vi "MGCC_FntStaMach_figureplot_main.vi"() -> ()   [LabVIEW 2016]
doc: "-----------------------------------------------------------------------------------------------------------------------\nCopyright <2019> <The University of Tennessee at Knoxville and the University of Tennessee Research Foundation>\nThis software is released under BSD-3 \nhttps://opensource.org/licenses/BSD-3-Clause \nAdditional license options available at https://utrf.tennessee.edu/industry/sample-agreements/\n-----------------------------------------------------------------------------------------------------------------------"
panel:
  out "Voltage difference1 14":cluster{dbl[], dbl[]}(graph)
  out "Voltage difference1 13":cluster{dbl[], dbl[]}(graph)
  out "Voltage difference1 11":cluster{dbl[], dbl[]}(graph)
  out "Voltage difference1 10":cluster{dbl[], dbl[]}(graph)
  out "Voltage difference1 9":cluster{dbl[], dbl[]}(graph)
  out "Voltage difference1 8":cluster{dbl[], dbl[]}(graph)
  out "Voltage difference1 7":cluster{dbl[], dbl[]}(graph)
  out "Voltage difference1 6":cluster{dbl[], dbl[]}(graph)
  out "Voltage difference1 5":cluster{dbl[], dbl[]}(graph)
  out "Voltage difference1 4":cluster{dbl[], dbl[]}(graph)
  out "Voltage difference1 3":cluster{dbl[], dbl[]}(graph)
  out "Voltage difference1 2":cluster{dbl[], dbl[]}(graph)
  out "Voltage phase":cluster{dbl[], dbl[]}[](graph)
  out "Voltage difference1":cluster{dbl[], dbl[]}(graph)
  # "Voltage"
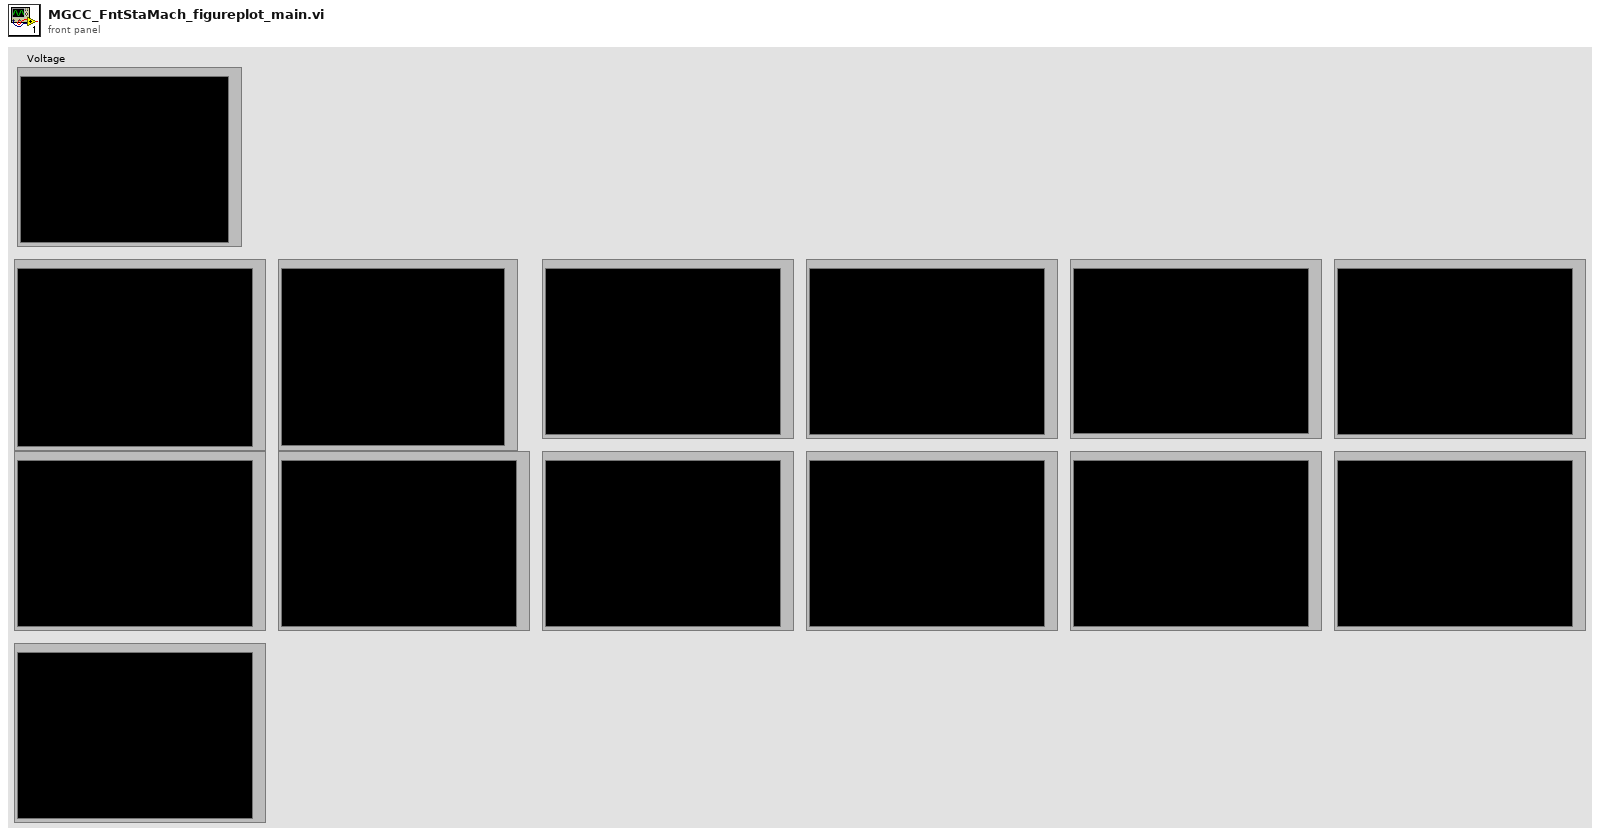
[diagram p1: front panel]
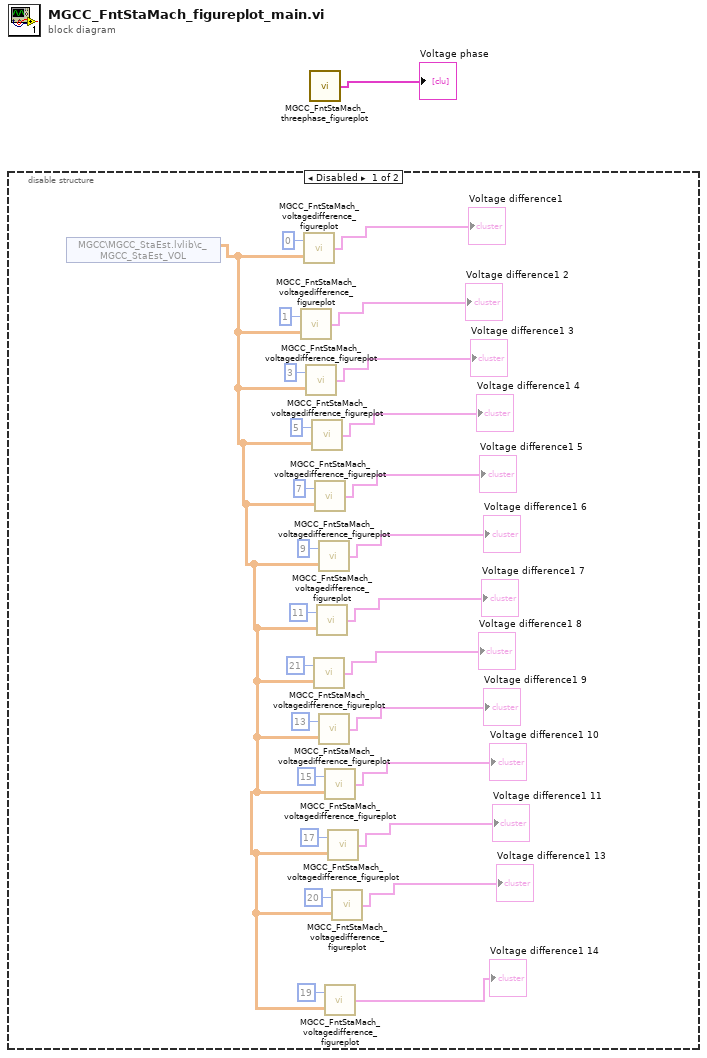
[diagram p0: block diagram]
diagram:
  n1 = disable-structure shown="Disabled" {
    frame Disabled {
      n2 = shared-variable "MGCC\\MGCC_StaEst.lvlib\\c_MGCC_StaEst_VOL"() -> (w3:cdb[][])  [unwired: 1 in, 1 out]
      n3 = call "MGCC_FntStaMach_voltagedifference_figureplot.vi"("array"=w3, "index (row)"=1) -> ("output cluster"=→"Voltage difference1 2":cluster{dbl[], dbl[]})
      n4 = call "MGCC_FntStaMach_voltagedifference_figureplot.vi"("array"=w3, "index (row)"=0) -> ("output cluster"=→"Voltage difference1":cluster{dbl[], dbl[]})
      n5 = call "MGCC_FntStaMach_voltagedifference_figureplot.vi"("array"=w3, "index (row)"=3) -> ("output cluster"=→"Voltage difference1 3":cluster{dbl[], dbl[]})
      n6 = call "MGCC_FntStaMach_voltagedifference_figureplot.vi"("array"=w3, "index (row)"=5) -> ("output cluster"=→"Voltage difference1 4":cluster{dbl[], dbl[]})
      n7 = call "MGCC_FntStaMach_voltagedifference_figureplot.vi"("array"=w3, "index (row)"=21) -> ("output cluster"=→"Voltage difference1 8":cluster{dbl[], dbl[]})
      n8 = call "MGCC_FntStaMach_voltagedifference_figureplot.vi"("array"=w3, "index (row)"=7) -> ("output cluster"=→"Voltage difference1 5":cluster{dbl[], dbl[]})
      n9 = call "MGCC_FntStaMach_voltagedifference_figureplot.vi"("array"=w3, "index (row)"=11) -> ("output cluster"=→"Voltage difference1 7":cluster{dbl[], dbl[]})
      n10 = call "MGCC_FntStaMach_voltagedifference_figureplot.vi"("array"=w3, "index (row)"=9) -> ("output cluster"=→"Voltage difference1 6":cluster{dbl[], dbl[]})
      n11 = call "MGCC_FntStaMach_voltagedifference_figureplot.vi"("array"=w3, "index (row)"=13) -> ("output cluster"=→"Voltage difference1 9":cluster{dbl[], dbl[]})
      n12 = call "MGCC_FntStaMach_voltagedifference_figureplot.vi"("array"=w3, "index (row)"=15) -> ("output cluster"=→"Voltage difference1 10":cluster{dbl[], dbl[]})
      n13 = call "MGCC_FntStaMach_voltagedifference_figureplot.vi"("array"=w3, "index (row)"=19) -> ("output cluster"=→"Voltage difference1 14":cluster{dbl[], dbl[]})
      n14 = call "MGCC_FntStaMach_voltagedifference_figureplot.vi"("array"=w3, "index (row)"=17) -> ("output cluster"=→"Voltage difference1 11":cluster{dbl[], dbl[]})
      n15 = call "MGCC_FntStaMach_voltagedifference_figureplot.vi"("array"=w3, "index (row)"=20) -> ("output cluster"=→"Voltage difference1 13":cluster{dbl[], dbl[]})
    }
    frame Enabled {
    }
  }
  n16 = call "MGCC_FntStaMach_threephase_figureplot.vi"() -> ("appended array"=→"Voltage phase":cluster{dbl[], dbl[]}[])
